vi "New Named Numeric Strings Binding.vi"(10 "NmdNum Refnum":refnum<vi>) -> (0 "error out":errorcluster, 3 "NamedNumericStringsBinding":refnum<class "NamedNumericStringsBinding.lvclass">)   [LabVIEW 2015, in "Transport.lvlib" / "NamedNumericStringsBinding.lvclass"]
doc: "<License>\nCopyright © 2017 Composed Systems, LLC | All rights reserved\nwww.composed.io\n\nAuthor: Ethan Stern <ethan.stern@composed.io>\n\nThis software is provided \"AS IS\" WITHOUT WARRANTIES, either express or implied, AND IS FOR EDUCATIONAL PURPOSES ONLY.\n</License>MVA Framework 1.0.4.16\nEthan Stern - Composed Systems\nCopyright (c) 2017, Composed Systems"
uses:
  NamedNumericStringsBinding.lvclass
  NamedNumericStringsBinding.lvclass/NamedNumericStringsBinding.ctl
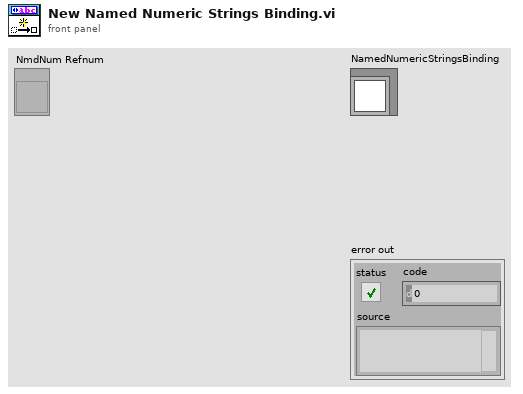
[diagram p1: front panel]
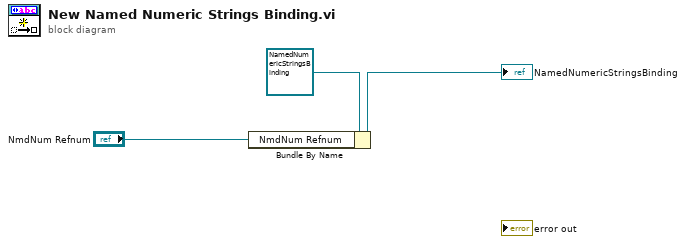
[diagram p0: block diagram]
diagram:
  n1 = Bundle By Name(cluster=refnum<class "NamedNumericStringsBinding.lvclass"> refnum ("TerminalReference in"), "NmdNum Refnum"="NmdNum Refnum") -> (→"NamedNumericStringsBinding":refnum<class "NamedNumericStringsBinding.lvclass">)
